vi "Becker-Hickl Read Single U16.vi"(8 "Error In":errorcluster, 10 "Default":u16, 11 "Bytes in":string) -> (0 "Error Out":errorcluster, 2 "U16":u16, 3 "Bytes out":string)   [LabVIEW 2021, in "Becker-Hickl Files.lvlib"]
uses:
  Becker-Hickl Files.lvlib
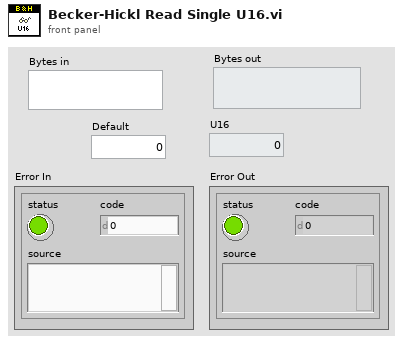
[diagram p1: front panel]
types:
  T1 = enum16{"big-endian, network order", "native, host order", "little-endian"}
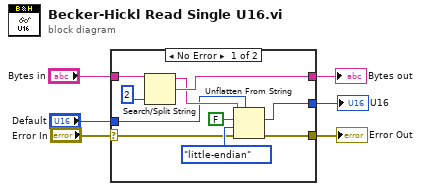
[diagram p0: block diagram]
diagram:
  n1 = case shown="No Error" "Error In" {
    selector: "Error In" -> [w9 w17]
    tunnel: [w16 _] -> w6
    tunnel: [w13 w18] -> w5
    tunnel: "Bytes in" -> [w15 w18]
    tunnel: [w8 w17] -> w2
    tunnel: "Default" -> [w7 _]
    frame No Error {
      n2 = Search/Split String(string=w15, offset (0)=2 ("index")) -> (substring before match=w10:string, match + rest of string=w13:string)  [unwired: 1 in, 1 out]
      n3 = Unflatten From String(type=w7, binary string=w10, data includes array or string size? (T)=FALSE, byte order (0:big-endian, network order)=T1."little-endian", error in (no error)=w9) -> (value=w16:u16, error out=w8:errorcluster)  [unwired: 1 out]
    }
    frame Error {
    }
  }
  "U16" <- w6
  "Bytes out" <- w5
  "Error Out" <- w2
